vi "Select Inheritance Location.vi"(8 "error in (no error)":errorcluster, 10 "NewVal":enum32{"Tree", "Path"}(ring), 11 "QControlWizard in":refnum<class "QControl Creation Wizard.lvclass">) -> (0 "error out":errorcluster, 3 "QControlWizard (dup)":refnum<class "QControl Creation Wizard.lvclass">)   [LabVIEW 2015, in "QControl Creation Wizard.lvclass"]
doc: "<b> </b> <b> </b>\n©2016 Q Software Innovations, LLC (QSI)\nwritten by Quentin Alldredge\nproduced in LabVIEW 2015\n\nsupport@qsoftwareinnovations.com\nwww.qsoftwareinnovations.com\n\nAll rights reserved.\n\nRedistribution and use in source and binary forms, with or without modification, are permitted provided that the following conditions are met:\n\n * Redistributions of source code must retain the above copyright notice, this list of conditions and the following disclaimer.\n * Redistributions in binary form must reproduce the above copyright notice, this list of conditions and the following disclaimer in the documentation and/or other materials provided with the distribution.\n * Neither the name of Q Software Innovations, LLC. nor the names of its contributors may be used to endorse or promote products derived from this software without specific prior written permission.\n\nTHIS SOFTWARE IS PROVIDED BY THE COPYRIGHT HOLDERS AND CONTRIBUTORS \"AS IS\" AND ANY EXPRESS OR IMPLIED WARRANTIES, INCLUDING, BUT NOT LIMITED TO, THE IMPLIED WARRANTIES OF MERCHANTABILITY AND FITNESS FOR A PARTICULAR PURPOSE ARE DISCLAIMED. IN NO EVENT SHALL THE COPYRIGHT OWNER OR CONTRIBUTORS BE LIABLE FOR ANY DIRECT, INDIRECT, INCIDENTAL, SPECIAL, EXEMPLARY, OR CONSEQUENTIAL DAMAGES (INCLUDING, BUT NOT LIMITED TO, PROCUREMENT OF SUBSTITUTE GOODS OR SERVICES; LOSS OF USE, DATA, OR PROFITS; OR BUSINESS INTERRUPTION) HOWEVER CAUSED AND ON ANY THEORY OF LIABILITY, WHETHER IN CONTRACT, STRICT LIABILITY, OR TORT (INCLUDING NEGLIGENCE OR OTHERWISE) ARISING IN ANY WAY OUT OF THE USE OF THIS SOFTWARE, EVEN IF ADVISED OF THE POSSIBILITY OF SUCH DAMAGE."
uses:
  QControl Creation Wizard.lvclass
  QControl Creation Wizard.lvclass/QControl Creation Wizard.ctl
  QControl Classes/TreeSelectionSingle/TreeSelectionSingle.lvclass
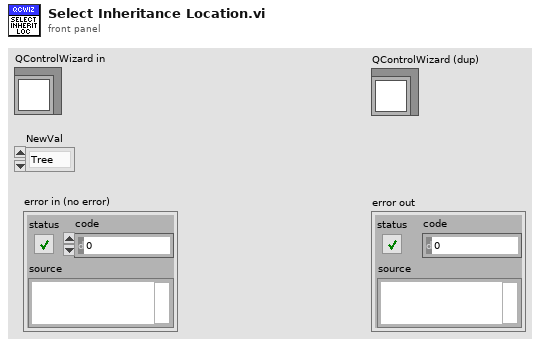
[diagram p1: front panel]
types:
  T1 = enum8{"Enabled", "Disabled", "Disabled and Grayed Out"}
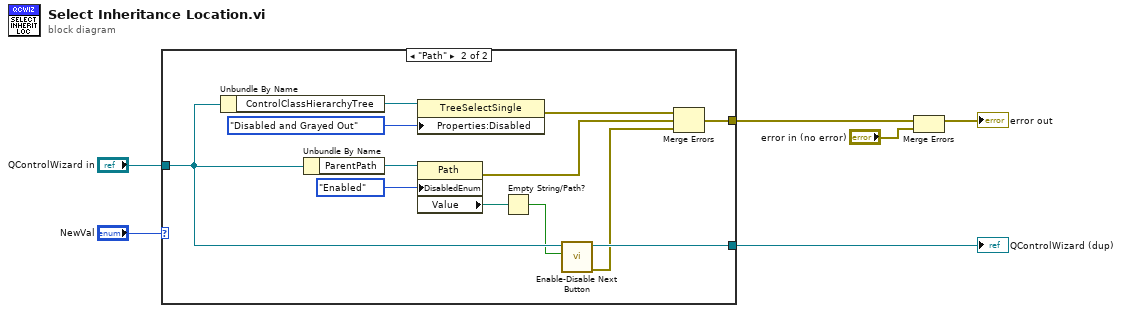
[diagram p0: block diagram]
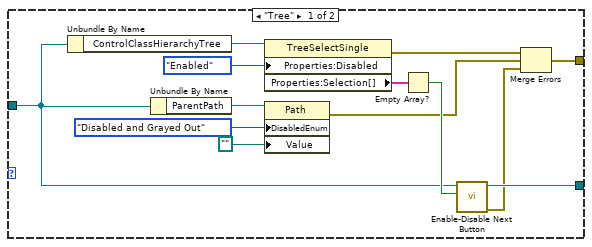
[diagram p2: hidden frame]
diagram:
  n1 = case shown="\"Path\"" "NewVal" {
    tunnel: "QControlWizard in" -> [w13 w26]
    tunnel: [w12 w24] -> w4
    tunnel: [w7 w20] -> w3
    frame "Tree" {
      n2 = Unbundle By Name(w13) -> ("ControlClassHierarchyTree"=w19:refnum<class "TreeSelectionSingle.lvclass">)
      n3 = Unbundle By Name(w13) -> ("ParentPath"=w17:refnum<vi>)
      n4 = property class="TreeSelectSingle"(reference=w19, "Properties:Disabled"=T1."Enabled" ("Disabled")) -> (error out=w10:errorcluster, "Properties:Selection[]"=w15:string[])  [unwired: 1 in, 1 out]
      n5 = property class="Path"(reference=w17, "DisabledEnum"=T1."Disabled and Grayed Out" ("Disabled"), "Value"=path "") -> (error out=w9:errorcluster)  [unwired: 1 in, 1 out]
      n6 = Empty Array?(array=w15) -> (empty?=w14:bool)
      n7 = call "Enable-Disable Next Button.vi"("Disable Next Button?"=w14, "QControlWizard in"=w13) -> ("error out"=w8:errorcluster, "QControlWizard (dup)"=w12:refnum<class "QControl Creation Wizard.lvclass">)  [unwired: 8 in]
      n8 = Merge Errors(w10, w9, w8) -> (w7:errorcluster)
    }
    frame "Path" {
      n9 = Unbundle By Name(w26) -> ("ControlClassHierarchyTree"=w31:refnum<class "TreeSelectionSingle.lvclass">)
      n10 = Unbundle By Name(w26) -> ("ParentPath"=w29:refnum<vi>)
      n11 = property class="TreeSelectSingle"(reference=w31, "Properties:Disabled"=T1."Disabled and Grayed Out" ("Disabled")) -> (error out=w23:errorcluster)  [unwired: 1 in, 1 out]
      n12 = property class="Path"(reference=w29, "DisabledEnum"=T1."Enabled" ("Disabled")) -> (error out=w22:errorcluster, "Value"=w27:path)  [unwired: 1 in, 1 out]
      n13 = Empty String/Path?(string/path=w27) -> (empty?=w25:bool)
      n14 = call "Enable-Disable Next Button.vi"("Disable Next Button?"=w25, "QControlWizard in"=w26) -> ("error out"=w21:errorcluster, "QControlWizard (dup)"=w24:refnum<class "QControl Creation Wizard.lvclass">)  [unwired: 8 in]
      n15 = Merge Errors(w23, w22, w21) -> (w20:errorcluster)
    }
  }
  "QControlWizard (dup)" <- w4
  n16 = Merge Errors(w3, "error in (no error)") -> (→"error out":errorcluster)
